vi "NI change inner param.vi"(8 "error in (no error)":errorcluster, 11 "NI in":refnum<class "NI.lvclass">) -> (0 "error out":errorcluster, 3 "NI out":refnum<class "NI.lvclass">)   [LabVIEW 2021, in "NI.lvlib" / "NI.lvclass"]
uses:
  NI.lvclass
  Channel Connection.ctl
  NI.lvclass/NI.ctl
panel:
  in  "Inner parameters":T2
  in  "OK Button":bool
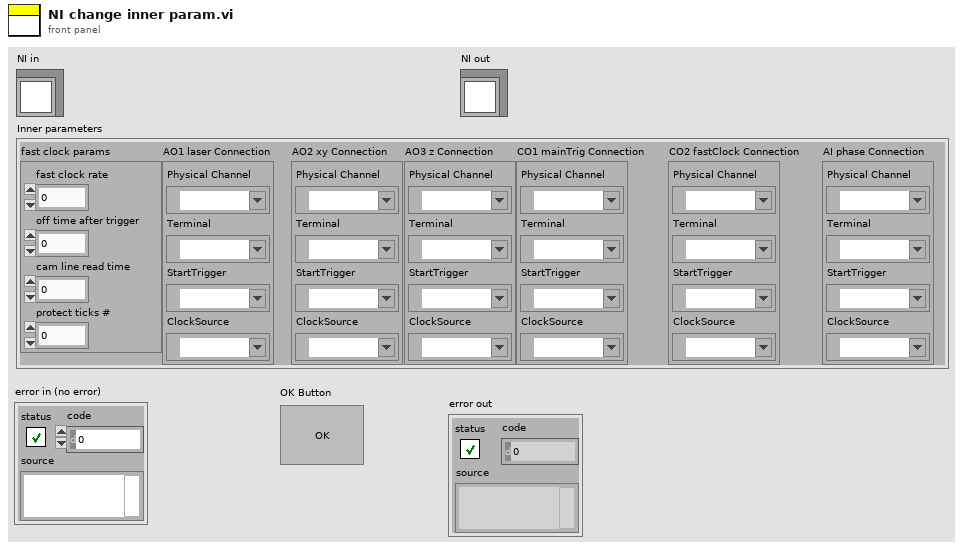
[diagram p1: front panel]
types:
  T1 = typedef "NI.lvlib/NI.lvclass/Channel Connection.ctl" = cluster{"Physical Channel":tag, "Terminal":tag, "StartTrigger":tag, "ClockSource":tag}
  T2 = cluster{"fast clock params":cluster{"fast clock rate":dbl, "off time after trigger":dbl, "cam line read time":dbl, "protect ticks #":dbl}, "AO1 laser Connection":T1, "AO2 xy Connection":T1, "AO3 z Connection":T1, "CO1 mainTrig Connection":T1, "CO2 fastClock Connection":T1, "AI phase Connection":T1}
  T3 = cluster{"fast clock params":cluster{"fast clock rate":dbl, "off time after trigger":dbl, "cam line read time":dbl, "protect ticks #":dbl}, "AO1 laser Connection":T1, "AO2 zy Connection":T1, "AO3 z Connection (deprecated)":T1, "CO1 mainTrig Connection":T1, "CO2 fastClock Connection":T1, "AI phase Connection":T1}
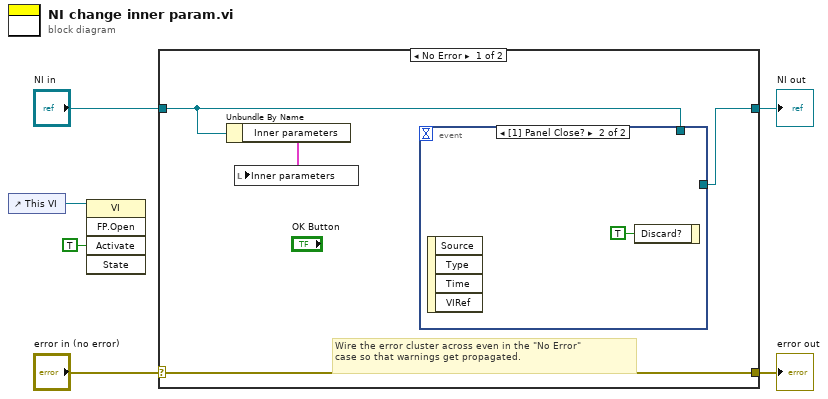
[diagram p0: block diagram]
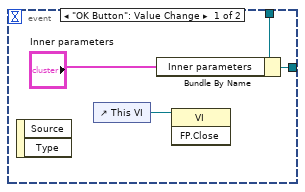
[diagram p2: hidden frame]
diagram:
  n1 = control-ref of="This VI"() -> (w1:refnum<vi>)
  n2 = invoke class="VI" method="FP.Open"(reference=w1, "Activate"=TRUE ("Activate?")) -> ()  [unwired: 3 in, 5 out]
  n3 = case shown="No Error" "error in (no error)" {
    selector: "error in (no error)" -> [w10 w17]
    tunnel: [w10 w17] -> w5
    tunnel: [w8 w16] -> w3
    tunnel: "NI in" -> [w9 w16]
    frame No Error {
      # "Wire the error cluster across even in the \"No Error\"\ncase so that warnings get propagated."
      n4 = Unbundle By Name(w9) -> ("Inner parameters"=w7:T3)
      n5 = local write "Inner parameters"(w7) -> ()
      n6 = event shown="[1] Panel Close?" {
        selector: _ -> [_ _]
        dyn-events: _ -> [_ _]
        timeout: _ -> [_ _]
        tunnel: w9 -> [w12 _]
        tunnel: [w11 _] -> w8
        event "OK Button": Value Change {
          n7 = event-data() -> ()  [unwired: 1 in, 2 out]
          n8 = control-ref of="This VI"() -> (w14:refnum<vi>)
          n9 = Bundle By Name(cluster=w12, "Inner parameters"="Inner parameters") -> (w11:refnum<class "NI.lvclass">)
          n10 = invoke class="VI" method="FP.Close"(reference=w14) -> ()  [unwired: 2 in, 3 out]
        }
        event Panel Close? {
          n11 = event-data() -> ()  [unwired: 1 in, 4 out]
          n12 = event-data("Discard?"=TRUE) -> ()  [unwired: 1 in, 1 out]
        }
      }
    }
    frame Error {
    }
  }
  "error out" <- w5
  "NI out" <- w3
